vi "Open read and close E&S emibin file.vi"(0 "file path":path, 11 "error in":errorcluster, 12 "File sub type(All)":u16=65535, 13 "Version(All)":u8=255) -> (8 "E&S records":T1[](array[typedef]), 10 "Numb records":i32, 15 "error out":errorcluster)   [LabVIEW 2011]
uses:
  emi Lib/System 01/0 - General/S&E reporting/Private/_emi_ S&E Message.ctl
  emi Lib/System 01/0 - General/S&E reporting/Private/_emi_ S&E Message type.ctl
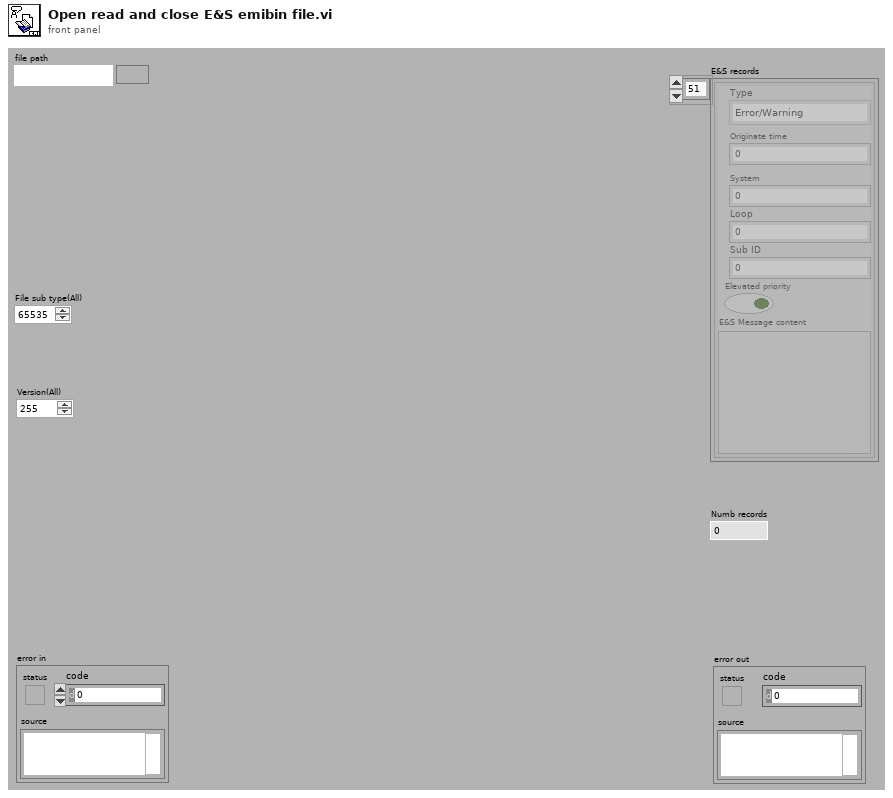
[diagram p1: front panel]
types:
  T1 = typedef "_emi_ S&E Message.ctl" = cluster{"Type":T2, "Originate time":dbl, "System":u8, "Loop":u16, "Sub ID":u16, "Elevated priority":bool, "E&S Message content":variant}
  T2 = typedef "_emi_ S&E Message type.ctl" = enum16{"Error/Warning", "Note", "Debug", "Event", "Alarm Analog", "Alarm Digital", "Annotation"}
  T3 = enum16{"big-endian, network order", "native, host order", "little-endian"}
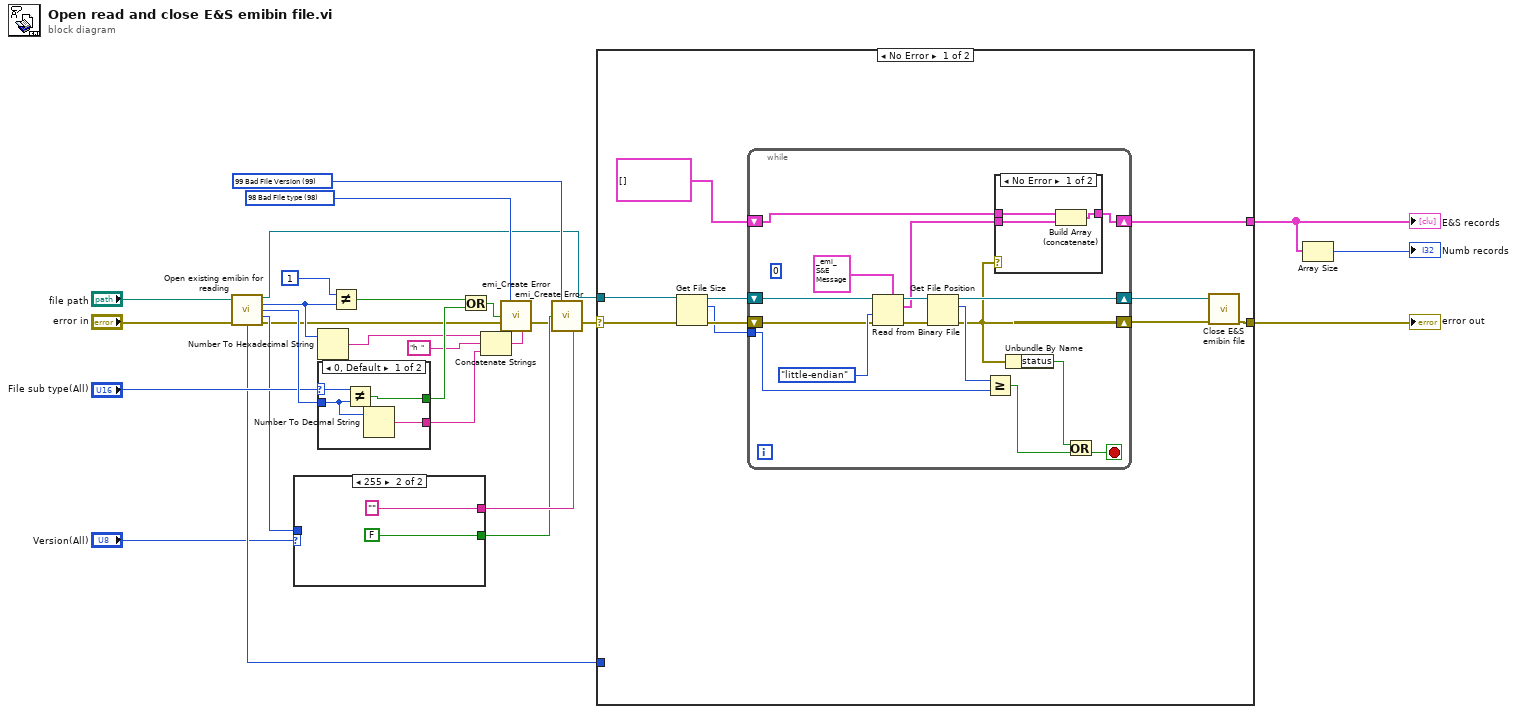
[diagram p0: block diagram]
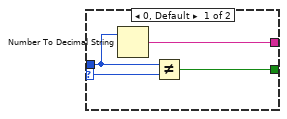
[diagram p2: hidden frame]
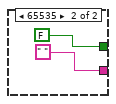
[diagram p3: hidden frame]
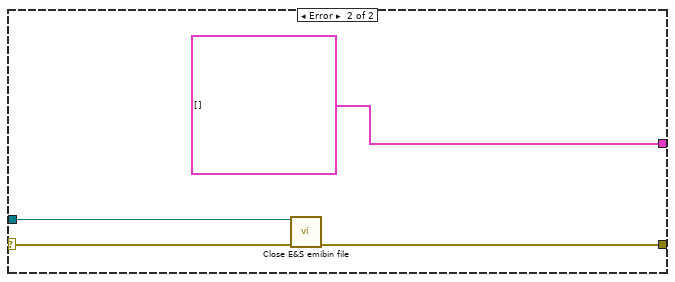
[diagram p5: hidden frame]
diagram:
  w14 = 99 items=["0 No Error"=0, "1 Invalid input parameter"=1, "6 Generic file IO "=6, "7 File not Found"=7, "35 Generic Pring Error"=35, "37 Device not Found"=37, "39 Device Unit Error"=39, "40 Could fot Open Device"=40, "42 Generic Error"=42, "52 Unknown Message"=52, "98 Bad File type"=98, "99 Bad File Version"=99, "100 Bad Data in File"=100, "1018 Unspecefied Error"=1018, "1041 Incorrect Password"=1041, "1043 Feature not in this version"=1043, "1109 Unsuported Data type"=1109, "1444 Did not close sucessfully"=1444] ("Error Code")
  w13 = 98 items=["0 No Error"=0, "1 Invalid input parameter"=1, "6 Generic file IO "=6, "7 File not Found"=7, "35 Generic Pring Error"=35, "37 Device not Found"=37, "39 Device Unit Error"=39, "40 Could fot Open Device"=40, "42 Generic Error"=42, "52 Unknown Message"=52, "98 Bad File type"=98, "99 Bad File Version"=99, "100 Bad Data in File"=100, "1018 Unspecefied Error"=1018, "1041 Incorrect Password"=1041, "1043 Feature not in this version"=1043, "1109 Unsuported Data type"=1109, "1444 Did not close sucessfully"=1444] ("Error Code")
  n1 = call "Open existing emibin for reading.vi"("file path"="file path", "error in (no error)"="error in") -> ("refnum out"=w1:refnum<file>, "File type Std"=w17:u8, "File type ID"=w26:u16, "File type Version"=w20:u8, "size (in bytes)"=w8:i64, "error out"=w11:errorcluster)  [unwired: 6 in, 2 out]
  n2 = case shown="255" "Version(All)" {
    selector: "Version(All)" -> [w28 _]
    tunnel: [w31 ""] -> w21
    tunnel: w20 -> [w30 _]
    tunnel: [w29 FALSE] -> w16
    frame 0, Default {
      n3 = Number To Decimal String(number=w30) -> (decimal integer string=w31:string)  [unwired: 1 in]
      n4 = Not Equal?(x=w30, y=w28) -> (x != y?=w29:bool)
    }
    frame 255 {
    }
  }
  n5 = Number To Hexadecimal String(2:w17) -> (0:w18:string)  [unwired: 1 in]
  n6 = case shown="0, Default" "File sub type(All)" {
    selector: "File sub type(All)" -> [w37 _]
    tunnel: [w34 " " ("string")] -> w23
    tunnel: [w36 FALSE] -> w25
    tunnel: w26 -> [w35 _]
    frame 0, Default {
      n7 = Not Equal?(x=w37, y=w35) -> (x != y?=w36:bool)
      n8 = Number To Decimal String(number=w35) -> (decimal integer string=w34:string)  [unwired: 1 in]
    }
    frame 65535 {
    }
  }
  n9 = Not Equal?(x=u8 1, y=w17) -> (x != y?=w15:bool)
  n10 = Or(x=w15, y=w25) -> (x .or. y?=w24:bool)
  n11 = Concatenate Strings(w18, "h  " ("string"), w23) -> (w3:string)
  n12 = call "emi_Create Error.vi"("Error Code"=w13, "Error(T)"=w24, "error in (no error)"=w11, "Append String(\"\")"=w3) -> ("error out"=w2:errorcluster)  [unwired: 11 in]
  n13 = call "emi_Create Error.vi"("Error Code"=w14, "Error(T)"=w16, "error in (no error)"=w2, "Append String(\"\")"=w21) -> ("error out"=w27:errorcluster)  [unwired: 11 in]
  n14 = case shown="No Error" w27 {
    selector: w27 -> [w48 w72]
    tunnel: [w49 w70] -> w7
    tunnel: w1 -> [w47 w71]
    tunnel: w8 -> [_ _]
    tunnel: [w41 T1[] []] -> w5
    frame No Error {
      n15 = Get File Size(file=w47, error in=w48) -> (refnum out=w46:refnum<file>, size (in bytes)=w42:i64, 0:w45:errorcluster)
      n16 = while {
        shift-right: [w50] -> w44
        shift-left: w45 -> [w60]
        shift-right: [w59] -> w43
        shift-left: w46 -> [w61]
        tunnel: w42 -> [w53]
        shift-right: [w52] -> w41
        shift-left: T1[] [] -> [w51]
        stop <- w55 stop-if-true
        (unwired) u32 0 ("unsigned 32bit integer")
        n17 = Read from Binary File(5:T1 {"Type"=enum."Error/Warning", "Originate time"=nan, "System"=0, "Loop"=9999, "Sub ID"=0, "Elevated priority"=FALSE, "E&S Message content"=variant} ("E&S Message"), 8:w60, 9:T3."little-endian" ("byte order (0:big-endian, network order)"), 11:w61) -> (0:w63:errorcluster, 2:w58:T1, 3:w62:refnum<file>)  [unwired: 2 in, 1 out]
        n18 = Get File Position(4:w63, 7:w62) -> (0:w50:errorcluster, 2:w56:i64, 3:w59:refnum<file>)
        n19 = Greater Or Equal?(x=w56, y=w53) -> (x >= y?=w57:bool)
        n20 = case shown="No Error" w50 {
          tunnel: w58 -> [w68 _]
          tunnel: [w67 w69] -> w52
          tunnel: w51 -> [w66 w69]
          frame No Error {
            n21 = Build Array (concatenate)(w66, w68) -> (w67:T1[])
          }
          frame Error {
          }
        }
        n22 = Unbundle By Name(w50) -> ("status"=w54:bool)
        n23 = Or(x=w54, y=w57) -> (x .or. y?=w55:bool)
      }
      n24 = call "Close E&S emibin file.vi"("refnum in"=w43, "error in (no error)"=w44) -> ("error out"=w49:errorcluster)  [unwired: 13 in]
    }
    frame Error {
      n25 = call "Close E&S emibin file.vi"("refnum in"=w71, "error in (no error)"=w72) -> ("error out"=w70:errorcluster)  [unwired: 13 in]
    }
  }
  "error out" <- w7
  "E&S records" <- w5
  n26 = Array Size(array=w5) -> (size(s)=→"Numb records":i32)
